vi "CRYSoundCard.vi"(8 "O_Name In":string[][](array[string]), 9 "I_Name In":string[][](array[string]), 10 "SoundCard In":T1={"Name"="", "Analog I/O"=0, "Digital I/O"=0, "Channels"=2, "Dig Dev ID"=1, "N ports"=3, "Interface"=0, "Dig I/O Ports"=[{"port #"=1, "width"=8, "direction"=0}, {"port #"=2, "width"=8, "direction"=0}, {"port #"=3, "width"=8, "direction"=0}], "Interf settings"=[], "N interfs"=3, "udev SNs"=[], "udev enable"=FALSE, "Channel Array"=[], "Cal sequence"="", "SelectedIn"=0, "SelectedOut"=0, "SelectedTab"=0, "State"=FALSE, "Help"="", "Advanced"=FALSE, "In Audio Driver"=0, "Out Audio Driver"=0} caption="Hardware" {"Channel Array"."Coupling" items=["Default"=-1, "RSE"=10083, "NRSE"=10078, "Differential"=10106, "Pseudodifferential"=12529]; "Channel Array"."term config" items=["Default"=-1, "RSE"=10083, "NRSE"=10078, "Differential"=10106, "Pseudodifferential"=12529]; "Channel Array"."Anti-aliasing Factor (%fs)" format="%.2f"}, 11 "Proper VI No In":i32) -> (0 "O_Name Out":string[][](array[string]), 1 "I_Name Out":string[][](array[string]))   [LabVIEW 2013]
uses:
  Typedef Control/CRYHardware.ctl
  Typedef Control/CRYHardware Channel Info.ctl
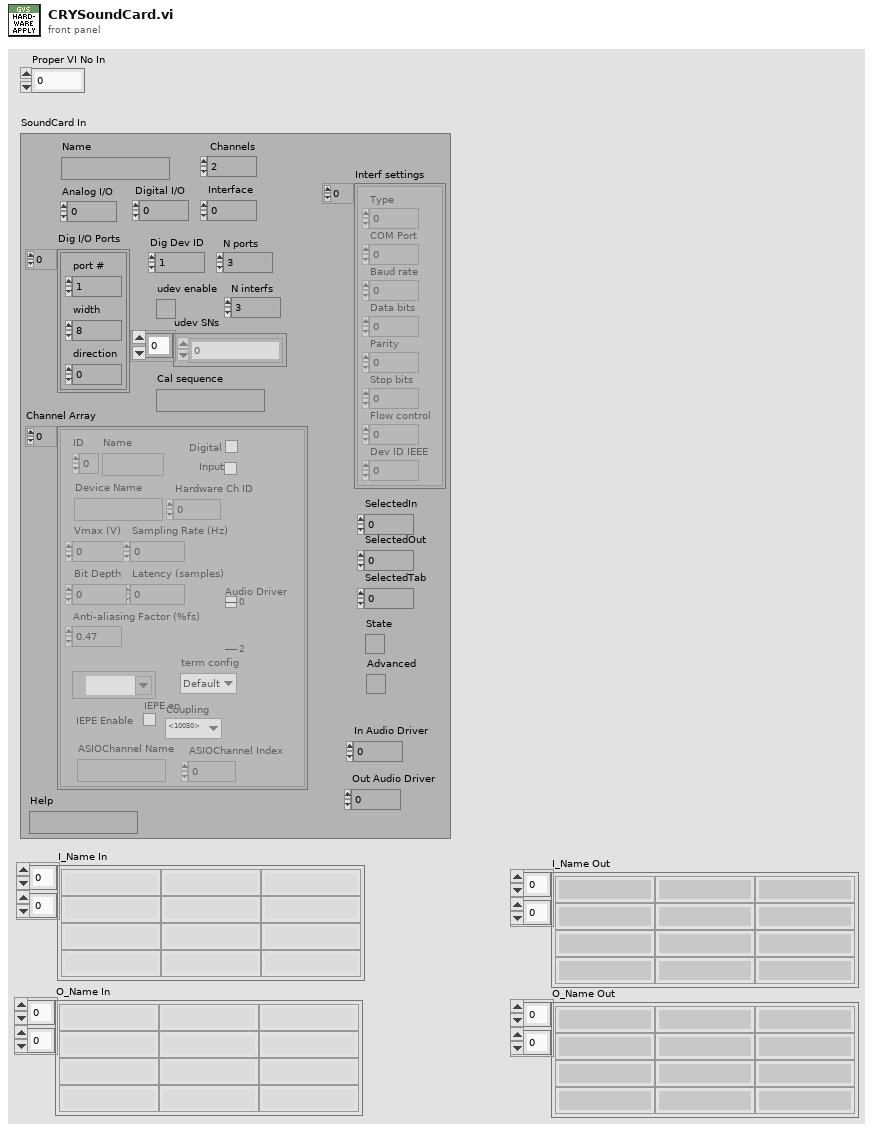
[diagram p1: front panel]
types:
  T1 = typedef "CRYHardware.ctl" = cluster{"Name":string, "Analog I/O":u16, "Digital I/O":u16, "Channels":u8, "Dig Dev ID":u8, "N ports":u8, "Interface":u32, "Dig I/O Ports":cluster{"port #":i16, "width":i16, "direction":i32}[], "Interf settings":cluster{"Type":u16, "COM Port":u8, "Baud rate":u32, "Data bits":u32, "Parity":u16, "Stop bits":u16, "Flow control":u16, "Dev ID IEEE":u8}[], "N interfs":i32, "udev SNs":i16[], "udev enable":bool, "Channel Array":T2[], "Cal sequence":string, "SelectedIn":u16, "SelectedOut":u16, "SelectedTab":u16, "State":bool, "Help":string, "Advanced":bool, "In Audio Driver":u16, "Out Audio Driver":u16}
  T2 = typedef "CRYHardware Channel Info.ctl" = cluster{"ID":i32, "Name":string, "Digital":bool, "Input":bool, "Device Name":string, "Hardware Ch ID":u8, "Vmax (V)":dbl, "Latency (samples)":dbl, "Sampling Rate (Hz)":u32, "Bit Depth":u32, "Anti-aliasing Factor (%fs)":sgl, "DAQmx Channel":tag, "term config":i32, "Coupling":i32, "IEPE en":bool, "ASIOChannel Name":string, "Audio Driver":u16, "ASIOChannel Index":u8}
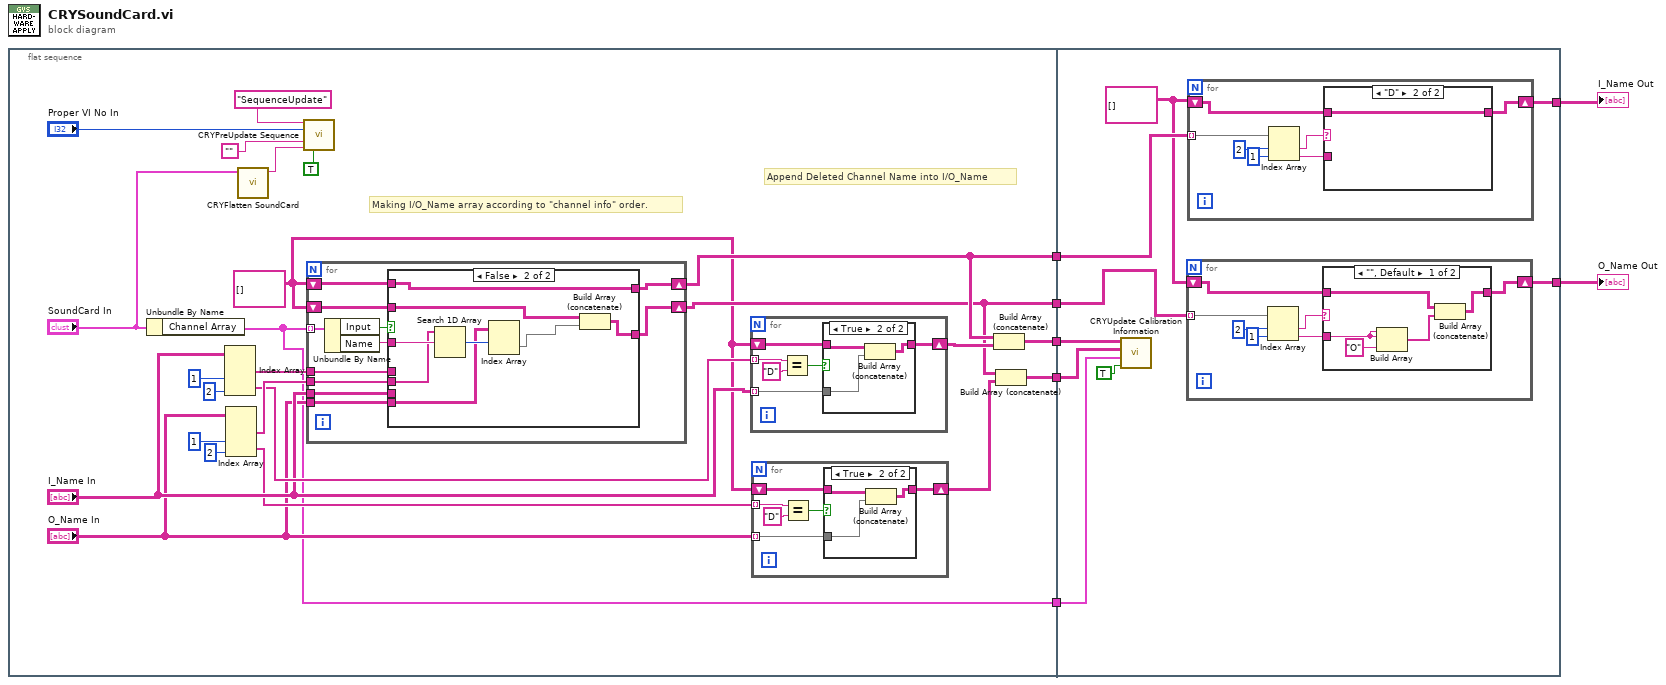
[diagram p0: block diagram]
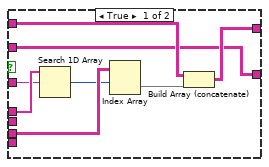
[diagram p4: hidden frame]
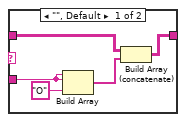
[diagram p6: hidden frame]
diagram:
  n1 = flat-sequence {
    tunnel: [w15] -> w5
    tunnel: [w9] -> w4
    tunnel: [w12] -> w3
    tunnel: [w11] -> w2
    tunnel: [w10] -> w1
    tunnel: [w86] -> w7
    tunnel: [w83] -> w6
    tunnel: w1 -> [w80]
    tunnel: w2 -> [w81]
    tunnel: w3 -> [w82]
    tunnel: w4 -> [w84]
    tunnel: w5 -> [w87]
    frame #0 {
      w8 = string[][] [] ("I_Name In")
      # "Append Deleted Channel Name into I/O_Name"
      # "Making I/O_Name array according to \"channel info\" order."
      n2 = Unbundle By Name("SoundCard In") -> ("Channel Array"=w10:T2[])
      n3 = Index Array(array="I_Name In", index (col) #1=1 ("disabled index (col)"), index (col) #2=2 ("index (col)")) -> (element #1=w20:string[], element #2=w19:string[])  [unwired: 2 in]
      n4 = Index Array(array="O_Name In", index (col) #1=1 ("disabled index (col)"), index (col) #2=2 ("index (col)")) -> (element #1=w23:string[], element #2=w17:string[])  [unwired: 2 in]
      n5 = call "CRYFlatten SoundCard.vi"("SoundCard"="SoundCard In") -> ("SoundCard flattened"=w29:string)  [unwired: 10 out]
      n6 = call "CRYPreUpdate Sequence.vi"("EventName"="SequenceUpdate", "Proper VI No"="Proper VI No In", "Project View Step Name Identifier Arg1"="", "Step flattened Arg2"=w29, "AllChangeFlg"=TRUE ("Name/Identifier")) -> ()  [unwired: 11 in]
      n7 = for {
        tunnel: w10 -> [w62] mode=indexing
        tunnel: w20 -> [w59]
        tunnel: "I_Name In" -> [w58]
        tunnel: "O_Name In" -> [w56]
        tunnel: w23 -> [w55]
        shift-right: [w57] -> w15
        shift-left: w8 -> [w54]
        shift-right: [w52] -> w9
        shift-left: w8 -> [w53]
        n8 = Unbundle By Name(w62) -> ("Input"=w61:bool, "Name"=w60:string)
        n9 = case shown="False" w61 {
          tunnel: w60 -> [w69 w78]
          tunnel: w59 -> [w70 _]
          tunnel: w58 -> [w68 _]
          tunnel: [w64 w71] -> w57
          tunnel: w56 -> [_ w76]
          tunnel: w55 -> [_ w75]
          tunnel: [w63 w73] -> w52
          tunnel: w54 -> [w65 w71]
          tunnel: w53 -> [w63 w72]
          frame True {
            n10 = Search 1D Array(1D array=w70, element=w69) -> (index of element=w67:i32)  [unwired: 1 in]
            n11 = Index Array(array=w68, index (row)=w67) -> (element=w66:string[])  [unwired: 1 in]
            n12 = Build Array (concatenate)(w65, w66) -> (w64:string[][])
          }
          frame False {
            n13 = Search 1D Array(1D array=w75, element=w78) -> (index of element=w77:i32)  [unwired: 1 in]
            n14 = Index Array(array=w76, index (row)=w77) -> (element=w74:string[])  [unwired: 1 in]
            n15 = Build Array (concatenate)(w72, w74) -> (w73:string[][])
          }
        }
      }
      n16 = for {
        tunnel: w19 -> [w45] mode=indexing
        tunnel: "I_Name In" -> [w44] mode=indexing
        shift-right: [w42] -> w14
        shift-left: w8 -> [w43]
        n17 = Equal?(x=w45, y="D") -> (x = y?=w46:bool)
        n18 = case shown="True" w46 {
          tunnel: w44 -> [_ w50]
          tunnel: w43 -> [w48 w51]
          tunnel: [w48 w49] -> w42
          frame False {
          }
          frame True {
            n19 = Build Array (concatenate)(w51, w50) -> (w49:string[][])
          }
        }
      }
      n20 = for {
        tunnel: w17 -> [w35] mode=indexing
        tunnel: "O_Name In" -> [w34] mode=indexing
        shift-right: [w32] -> w13
        shift-left: w8 -> [w33]
        n21 = Equal?(x=w35, y="D") -> (x = y?=w36:bool)
        n22 = case shown="True" w36 {
          tunnel: w34 -> [_ w40]
          tunnel: w33 -> [w38 w41]
          tunnel: [w38 w39] -> w32
          frame False {
          }
          frame True {
            n23 = Build Array (concatenate)(w41, w40) -> (w39:string[][])
          }
        }
      }
      n24 = Build Array (concatenate)(w15, w14) -> (w12:string[][])
      n25 = Build Array (concatenate)(w9, w13) -> (w11:string[][])
    }
    frame #1 {
      w85 = string[][] []
      n26 = call "CRYUpdate Calibration Information.vi"("From Hardware?"=TRUE, "Hardware Channel Array"=w80, "O_Name In"=w81, "I_Name In"=w82) -> ()  [unwired: 8 out]
      n27 = for {
        tunnel: w84 -> [w92] mode=indexing
        shift-right: [w88] -> w83
        shift-left: w85 -> [w89]
        n28 = Index Array(array=w92, index #1=2 ("index"), index #2=1 ("index")) -> (element #1=w90:string, element #2=w91:string)
        n29 = case shown="\"\", Default" w90 {
          tunnel: w91 -> [w98 _]
          tunnel: w89 -> [w97 w100]
          tunnel: [w95 w100] -> w88
          frame "", Default {
            n30 = Build Array(w98, w98, "O" ("element")) -> (w96:string[])
            n31 = Build Array (concatenate)(w97, w96) -> (w95:string[][])
          }
          frame "D" {
          }
        }
      }
      n32 = for {
        tunnel: w87 -> [w105] mode=indexing
        shift-right: [w101] -> w86
        shift-left: w85 -> [w102]
        n33 = Index Array(array=w105, index #1=2 ("index"), index #2=1 ("index")) -> (element #1=w103:string, element #2=w104:string)
        n34 = case shown="\"D\"" w103 {
          tunnel: w104 -> [w111 _]
          tunnel: w102 -> [w110 w113]
          tunnel: [w108 w113] -> w101
          frame "", Default {
            n35 = Build Array(w111, w111, "O" ("element")) -> (w109:string[])
            n36 = Build Array (concatenate)(w110, w109) -> (w108:string[][])
          }
          frame "D" {
          }
        }
      }
    }
  }
  "I_Name Out" <- w7
  "O_Name Out" <- w6
